vi "http 501 not implemented error.vi"(11 "application request in":T3) -> (3 "application request out":T1)   [LabVIEW 2013]
uses:
  http request.ctl
  http method.ctl
  http response.ctl
  http response packet type.ctl
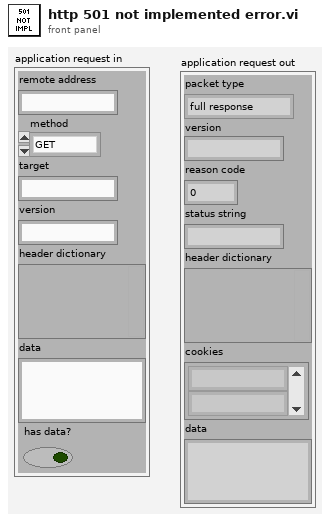
[diagram p1: front panel]
types:
  T1 = typedef "http response.ctl" = cluster{"packet type":T2, "version":string, "reason code":u16, "status string":string, "header dictionary":variant, "cookies":string[], "data":string}
  T2 = typedef "http response packet type.ctl" = enum16{"full response", "header only", "data only", "last data"}
  T3 = typedef "http request.ctl" = cluster{"remote address":string, "method":T4, "target":string, "version":string, "header dictionary":variant, "data":string, "has data?":bool}
  T4 = typedef "http method.ctl" = enum16{"GET", "POST", "PUT", "DELETE", "HEAD", "OPTIONS", "upgrade"}
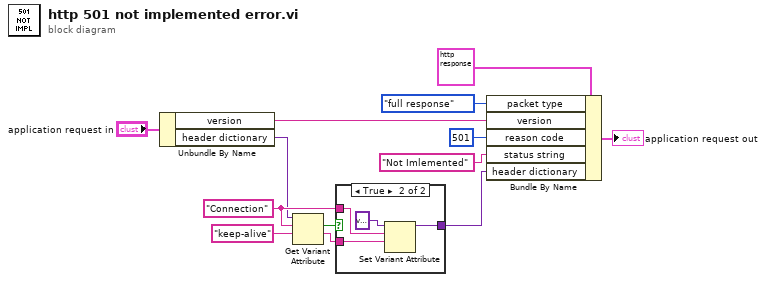
[diagram p0: block diagram]
diagram:
  w10 = "Connection" ("name")
  n1 = Unbundle By Name("application request in") -> ("version"=w6:string, "header dictionary"=w7:variant)
  n2 = Get Variant Attribute(Variant=w7, name=w10, default value (empty Variant)="keep-alive" ("name")) -> (found=w2:bool, value=w9:string)  [unwired: 1 in, 2 out]
  n3 = case shown="True" w2 {
    tunnel: [_ w17] -> w11
    tunnel: w10 -> [_ w16]
    tunnel: w9 -> [_ w15]
    frame False {
    }
    frame True {
      n4 = Set Variant Attribute(Variant=variant ("variant"), name=w16, value=w15) -> (Variant out=w17:variant)  [unwired: 1 in, 2 out]
    }
  }
  n5 = Bundle By Name(cluster=T1 {"packet type"=enum."full response", "version"="", "reason code"=0, "status string"="", "header dictionary"=variant, "cookies"=[], "data"=""} ("application request"), "packet type"=http_response_packet_type."full response", "version"=w6, "reason code"=u16 501, "status string"="Not Imlemented", "header dictionary"=w11) -> (→"application request out":T1)
